vi "Get Wfm Refs.vi"(8 "Error in":errorcluster, 10 "Scaling Enabled?":bool=TRUE, 11 "Device Ref in":T2 format="%.0x") -> (0 "Error out":errorcluster, 1 "Results Wfm Data Refs":T1[](array[typedef]), 2 "Source Wfm Data Refs":T1[](array[typedef]), 3 "Device Ref out":T2=18446744073709551615 format="%.0x")   [LabVIEW 2023, in "Waveform-Processing-Custom-Device System Explorer.lvlib"]
uses:
  Waveform-Processing-Custom-Device System Explorer.lvlib
  <vilib>/NI VeriStand/Custom Device API/Custom Device Item Ref.ctl
  <vilib>/NI VeriStand/Custom Device API/Waveform Data Reference.ctl
  Shared/Constants.vi
  <vilib>/NI VeriStand/Custom Device API/Get Item Property (Dependent Node Pointer).vi
  <vilib>/NI VeriStand/Custom Device API/Custom Device API.lvlib
  Shared/Waveform-Processing-Custom-Device Shared.lvlib
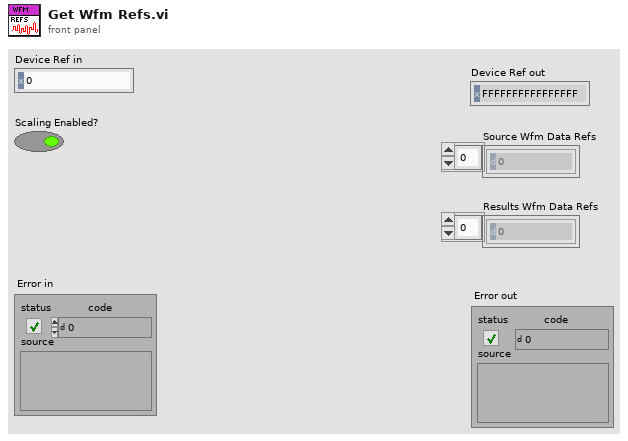
[diagram p1: front panel]
types:
  T1 = typedef "Custom Device API.lvlib/Waveform Data Reference.ctl" = i32
  T2 = typedef "Custom Device API.lvlib/Custom Device Item Ref.ctl" = u64
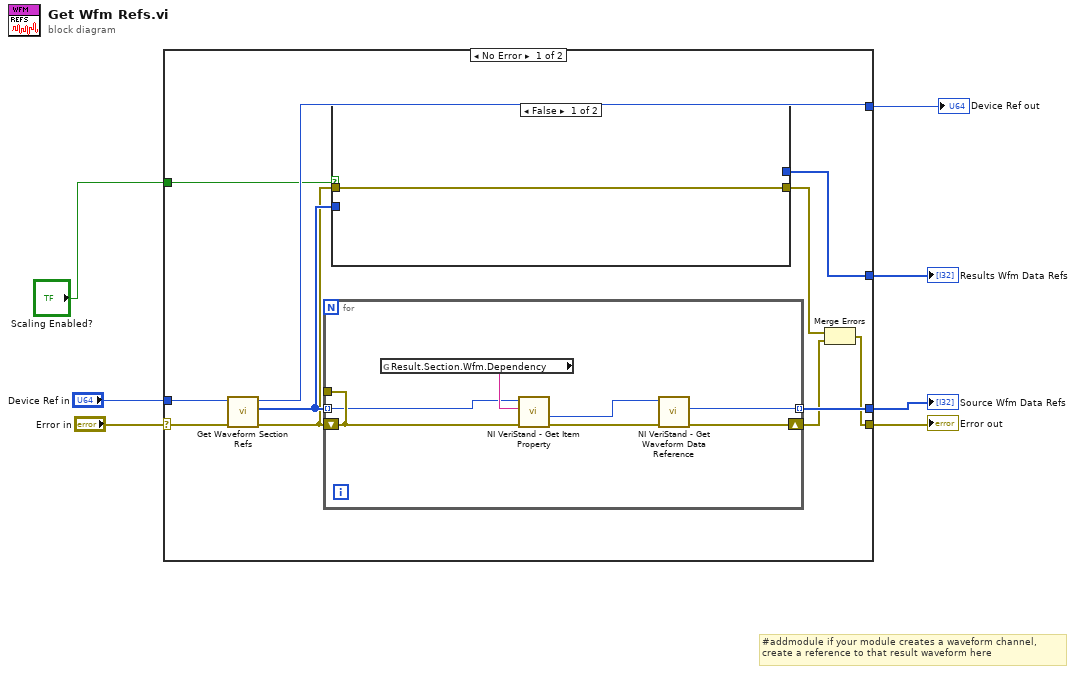
[diagram p0: block diagram]
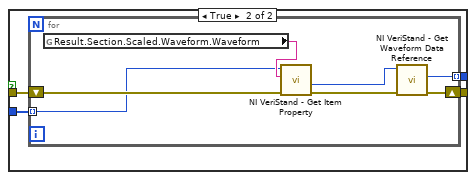
[diagram p2: hidden frame]
diagram:
  # "#addmodule if your module creates a waveform channel,\ncreate a reference to that result waveform here"
  n1 = case shown="No Error" "Error in" {
    selector: "Error in" -> [w18 w39]
    tunnel: [w13 w39] -> w6
    tunnel: "Device Ref in" -> [w17 w38]
    tunnel: [w16 w38] -> w4
    tunnel: [w15 _] -> w3
    tunnel: [w12 _] -> w2
    tunnel: "Scaling Enabled?" -> [w8 _]
    frame No Error {
      n2 = call "Get Waveform Section Refs.vi"("Error in"=w18, "Device Ref in"=w17) -> ("Error out"=w10:errorcluster, "Result Section Refs"=w14:T2[], "Device Ref out"=w16:T2)  [unwired: 7 in]
      n3 = for {
        tunnel: w14 -> [w32] mode=indexing
        tunnel: [w34] -> w15 mode=indexing
        shift-right: [w31] -> w9
        shift-left: w10 -> [w33]
        tunnel: [w33] -> _
        n4 = global read "Constants.vi" "Result.Section.Wfm.Dependency"() -> (w37:string)
        n5 = call-poly <vilib>:"NI VeriStand - Get Item Property.vi"("error in (no error)"=w33, "Property Name"=w37, "Item Ref in"=w32) -> ("error out"=w36:errorcluster, "Dependent Node Ref"=w35:T2)  [unwired: 5 in, 2 out]
        n6 = call <vilib>:"NI VeriStand - Get Waveform Data Reference.vi"("error in (no error)"=w36, "Waveform Ref in"=w35) -> ("error out"=w31:errorcluster, "Waveform Data Reference"=w34:T1)  [unwired: 7 in, 1 out]
      }
      n7 = case shown="False" w8 {
        tunnel: w14 -> [_ w23]
        tunnel: [_ w22] -> w12
        tunnel: [w19 w21] -> w11
        tunnel: w10 -> [w19 w20]
        frame False {
        }
        frame True {
          n8 = for {
            tunnel: w23 -> [w24] mode=indexing
            tunnel: [w27] -> w22 mode=indexing
            shift-right: [w28] -> w21
            shift-left: w20 -> [w26]
            n9 = global read "Constants.vi" "Result.Section.Scaled.Waveform.Waveform"() -> (w25:string)
            n10 = call-poly <vilib>:"NI VeriStand - Get Item Property.vi"("error in (no error)"=w26, "Property Name"=w25, "Item Ref in"=w24) -> ("error out"=w30:errorcluster, "Dependent Node Ref"=w29:T2)  [unwired: 5 in, 2 out]
            n11 = call <vilib>:"NI VeriStand - Get Waveform Data Reference.vi"("error in (no error)"=w30, "Waveform Ref in"=w29) -> ("error out"=w28:errorcluster, "Waveform Data Reference"=w27:T1)  [unwired: 7 in, 1 out]
          }
        }
      }
      n12 = Merge Errors(w11, w9) -> (w13:errorcluster)
    }
    frame Error {
    }
  }
  "Error out" <- w6
  "Device Ref out" <- w4
  "Source Wfm Data Refs" <- w3
  "Results Wfm Data Refs" <- w2
